vi "cm to in.vi"(5 "Centimeter":dbl) -> (2 "Inch":dbl)   [LabVIEW 2013]
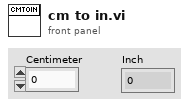
[diagram p1: front panel]
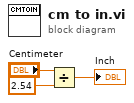
[diagram p0: block diagram]
diagram:
  n1 = Divide(x="Centimeter", y=2.54) -> (x/y=→"Inch":dbl)
